vi "Clear Merged Errors.vi"(0 "Export in":refnum<class "Export.lvclass">, 11 "error in (no error)":errorcluster) -> (4 "Export out":refnum<class "Export.lvclass">, 6 "Cleared Error":errorcluster, 15 "error out":errorcluster)   [LabVIEW 2017, in "CL_G3_VIComponentBuilder.lvlib" / "Export.lvclass"]
doc: "Clears the error status for this export."
uses:
  Export.lvclass
  Export.lvclass/Export.ctl
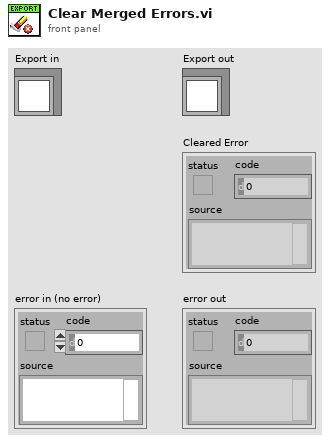
[diagram p1: front panel]
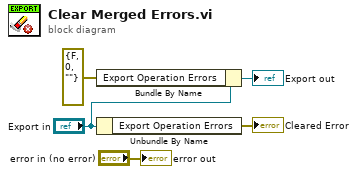
[diagram p0: block diagram]
diagram:
  n1 = Bundle By Name(cluster="Export in", "Export Operation Errors"=errorcluster {"status"=FALSE, "code"=0, "source"=""}) -> (→"Export out":refnum<class "Export.lvclass">)
  n2 = Unbundle By Name("Export in") -> ("Export Operation Errors"=→"Cleared Error":errorcluster)
  "error out" <- "error in (no error)"
